vi "gatherdata_backup.vi"() -> ()   [LabVIEW 2011]
uses:
  <vilib>/FPGAPlugInAG/sbRIO-9606/niLvFpga_Open_sbRIO-9606.vi
  <vilib>/rvi/interface/common/dynamic/niFpgaDynamicAddResources.vi
  <vilib>/Utility/error.llb/Error Cluster From Error Code.vi
  <vilib>/rvi/errors/niLvFpgaAdjustHostInterfaceError.vi
  <vilib>/rvi/interface/nirviOpenFPGA/nirviOpenFPGA.xnode
  labview/FPGA Bitfiles/natcar_FPGATarget_Top-Level_610FB000.lvbitx
  <vilib>/rvi/interface/nirviReadWriteControl/nirviReadWriteControl.xnode
  NiFpgaLv.dll
  <vilib>/rvi/interface/Simulation/niFpgaSimulationCallBeginRW.vi
panel:
  in  "stop":bool
  in  "Save Path and Filename":path
  out "AI7":u16
  out "AI6":u16
  out "AI5":u16
  out "AI4":u16
  out "AI3":u16
  out "AI2":u16
  out "AI1":u16
  out "AI0":u16
  in  "#pts to avg":dbl=100000.0
  out "Waiting":bool
  out "Saving\nData":bool
  out "Getting\nData":bool
  in  "distance":dbl
  in  "Record":bool
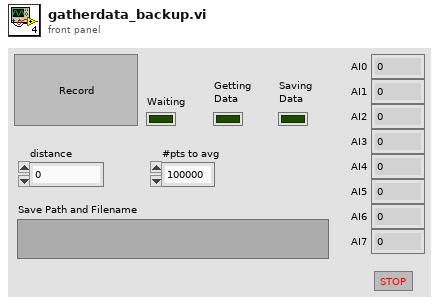
[diagram p1: front panel]
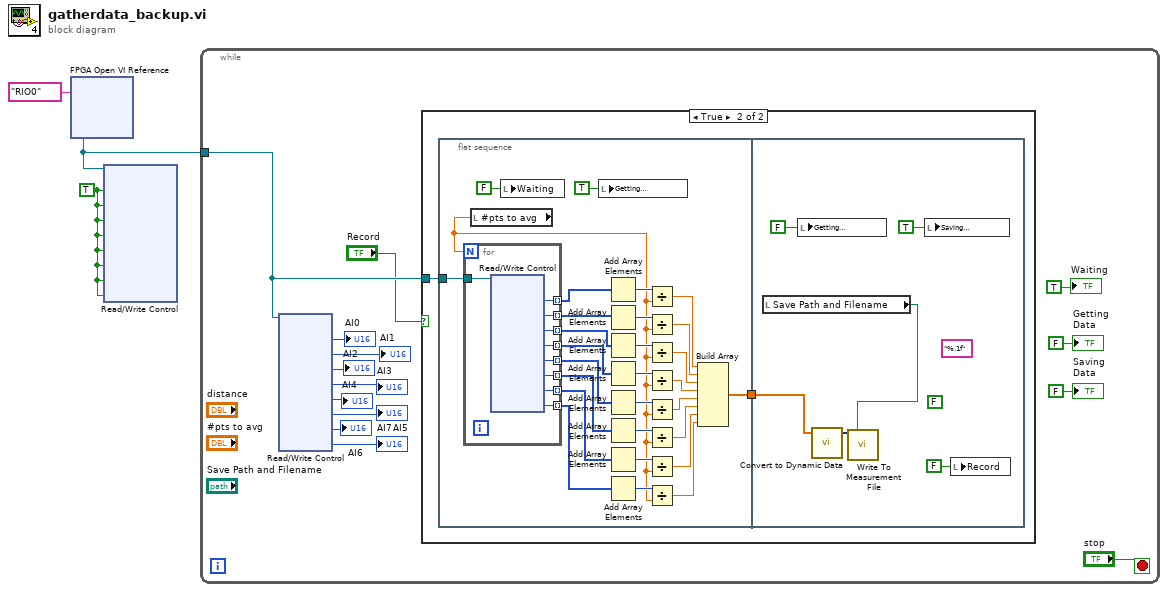
[diagram p0: block diagram]
diagram:
  w3 = TRUE ("Enable AI0")
  n1 = xnode "FPGA Open VI Reference"("resource name"=tag "RIO0") -> ("FPGA VI Reference Out"=w1:refnum<k20>)  [unwired: 1 in, 1 out]
  n2 = xnode "Read/Write Control"("FPGA VI Reference In"=w1, "Enable AI0"=w3, "Enable AI1"=w3, "Enable AI2"=w3, "Enable AI3"=w3, "Enable AI4"=w3, "Enable AI5"=w3, "Enable AI6"=w3, "Enable AI7"=w3) -> ()  [unwired: 1 in, 2 out]
  n3 = while {
    tunnel: w1 -> [w5]
    stop <- "stop" stop-if-true
    n4 = xnode "Read/Write Control"("FPGA VI Reference In"=w5) -> ("AI0"=→"AI0":u16, "AI1"=→"AI1":u16, "AI2"=→"AI2":u16, "AI3"=→"AI3":u16, "AI4"=→"AI4":u16, "AI5"=→"AI5":u16, "AI6"=→"AI6":u16, "AI7"=→"AI7":u16)  [unwired: 1 in, 2 out]
    n5 = case shown="True" "Record" {
      tunnel: w5 -> [_ w18]
      frame False {
      }
      frame True {
        n6 = flat-sequence {
          tunnel: [w21] -> w19
          tunnel: w18 -> [w20]
          tunnel: w19 -> [w58]
          frame #0 {
            n7 = local read "#pts to avg"() -> (w30:dbl)
            n8 = for {
              N: w30 -> [_]
              tunnel: [w57] -> w39 mode=indexing
              tunnel: [w56] -> w38 mode=indexing
              tunnel: [w55] -> w37 mode=indexing
              tunnel: [w54] -> w35 mode=indexing
              tunnel: [w53] -> w36 mode=indexing
              tunnel: [w52] -> w34 mode=indexing
              tunnel: [w51] -> w33 mode=indexing
              tunnel: [w50] -> w31 mode=indexing
              tunnel: w20 -> [w49]
              n9 = xnode "Read/Write Control"("FPGA VI Reference In"=w49) -> ("AI0"=w57:u16, "AI1"=w56:u16, "AI2"=w55:u16, "AI3"=w53:u16, "AI4"=w54:u16, "AI5"=w52:u16, "AI6"=w51:u16, "AI7"=w50:u16)  [unwired: 1 in, 2 out]
            }
            n10 = local write "Waiting"(FALSE ("Waiting")) -> ()
            n11 = local write "Getting\nData"(TRUE ("Getting\nData")) -> ()
            n12 = Add Array Elements(numeric array=w39) -> (sum=w46:u16)
            n13 = Add Array Elements(numeric array=w38) -> (sum=w45:u16)
            n14 = Add Array Elements(numeric array=w37) -> (sum=w44:u16)
            n15 = Add Array Elements(numeric array=w36) -> (sum=w43:u16)
            n16 = Add Array Elements(numeric array=w35) -> (sum=w42:u16)
            n17 = Add Array Elements(numeric array=w34) -> (sum=w41:u16)
            n18 = Add Array Elements(numeric array=w33) -> (sum=w40:u16)
            n19 = Add Array Elements(numeric array=w31) -> (sum=w32:u16)
            n20 = Divide(x=w46, y=w30) -> (x/y=w29:dbl)
            n21 = Divide(x=w45, y=w30) -> (x/y=w28:dbl)
            n22 = Divide(x=w44, y=w30) -> (x/y=w27:dbl)
            n23 = Divide(x=w43, y=w30) -> (x/y=w26:dbl)
            n24 = Divide(x=w42, y=w30) -> (x/y=w22:dbl)
            n25 = Divide(x=w41, y=w30) -> (x/y=w23:dbl)
            n26 = Divide(x=w40, y=w30) -> (x/y=w24:dbl)
            n27 = Divide(x=w32, y=w30) -> (x/y=w25:dbl)
            n28 = Build Array(w29, w28, w27, w26, w22, w23, w24, w25) -> (w21:dbl[])
          }
          frame #1 {
            (unwired) "%.1f" ("format (%.3f)")
            (unwired) FALSE ("append to file? (new file:F)")
            n29 = local read "Save Path and Filename"() -> (w60:path)
            n30 = local write "Getting\nData"(FALSE ("Getting\nData")) -> ()
            n31 = call "Convert to Dynamic Data"("Array"=w58) -> ("Dynamic Data Type"=w59:dynamicdata)  [unwired: 3 in]
            n32 = call "Write To Measurement File"("Signals"=w59, "Filename"=w60) -> ()  [unwired: 15 in, 3 out]
            n33 = local write "Saving\nData"(TRUE ("Getting\nData")) -> ()
            n34 = local write "Record"(FALSE ("Record")) -> ()
          }
        }
      }
    }
    "Getting\nData" <- FALSE ("Getting\nData")
    "Saving\nData" <- FALSE ("Saving\nData")
    "Waiting" <- TRUE ("Waiting")
  }
